vi "Update Lower Value.vi"(1 "Blue":cluster{"Lower value":i32, "Upper value":i32}, 2 "Numeric":dbl) -> (0 "Blue 2":cluster{"Lower value":i32, "Upper value":i32})   [LabVIEW 2010]
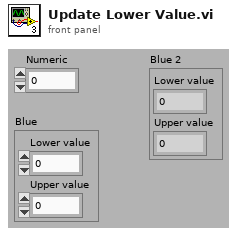
[diagram p1: front panel]
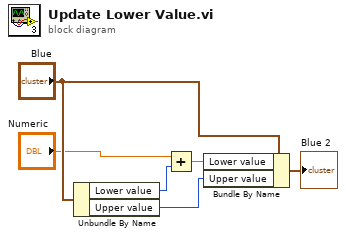
[diagram p0: block diagram]
diagram:
  n1 = Unbundle By Name("Blue") -> ("Lower value"=w3:i32, "Upper value"=w2:i32)
  n2 = Add(x="Numeric", y=w3) -> (x+y=w4:dbl)
  n3 = Bundle By Name(cluster="Blue", "Lower value"=w4, "Upper value"=w2) -> (→"Blue 2":cluster{"Lower value":i32, "Upper value":i32})
